vi "Error Code to Error Cluster.vi"(5 "is warning? (False)":bool, 7 "show call chain? (False)":bool, 8 "Error In":errorcluster, 10 "Error Message":string, 11 "CS++Error":T1 items=["No Error"=0, "Object configuration data not found"=5000]) -> (0 "Error Out":errorcluster)   [LabVIEW 2013, in "CS++Base.lvlib"]
uses:
  CS++Base.lvlib
  Error Definition.ctl
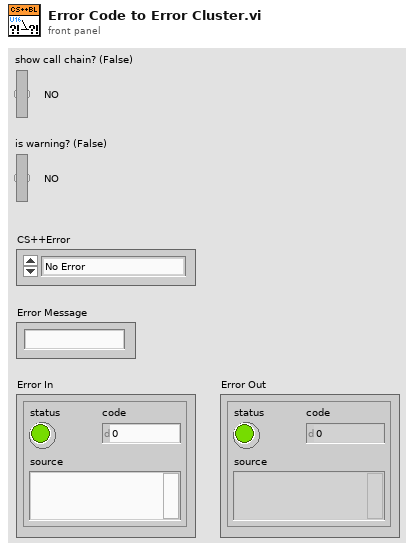
[diagram p1: front panel]
types:
  T1 = typedef "CS++Base.lvlib/Error Definition.ctl" = u16
  T2 = typedef "LVStringsAndValuesArrayTypeDef_U16.ctl" = cluster{"String":string, "Value":u16}[]
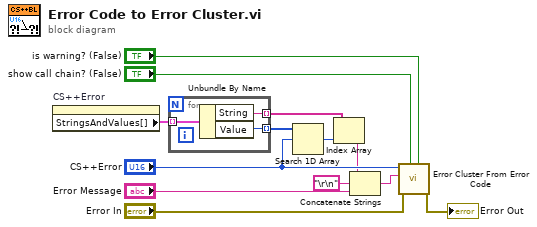
[diagram p0: block diagram]
diagram:
  n1 = property on="CS++Error" class="Ring (strict)"() -> ("StringsAndValues[]"=w11:T2)  [unwired: 2 in, 2 out]
  n2 = for {
    tunnel: w11 -> [w16] mode=indexing
    tunnel: [w15] -> w8 mode=indexing
    tunnel: [w14] -> w10 mode=indexing
    n3 = Unbundle By Name(w16) -> ("String"=w15:string, "Value"=w14:u16)
  }
  n4 = Search 1D Array(1D array=w10, element="CS++Error") -> (index of element=w7:i32)  [unwired: 1 in]
  n5 = Index Array(array=w8, index=w7) -> (element=w6:string)
  n6 = Concatenate Strings(w6, "\r\n", "Error Message") -> (w3:string)
  n7 = call <vilib>:"Error Cluster From Error Code.vi"("is warning? (False)"="is warning? (False)", "show call chain? (False)"="show call chain? (False)", "error in (no error)"="Error In", "error message (\"\")"=w3, "error code (0)"="CS++Error") -> ("error out"=→"Error Out":errorcluster)  [unwired: 4 in]
